vi "FTW-Container-Array-ReplaceSubset.vi"(0 "FTW-Container In":refnum<class "FTW-Container.lvclass">, 7 "Array Elements":refnum<class "FTW-Container.lvclass">[](array[class]), 9 "Index":i32, 11 "error in":errorcluster) -> (4 "FTW-Container Out":refnum<class "FTW-Container.lvclass">, 15 "error out":errorcluster)   [LabVIEW 2015, in "FTW-Container.lvclass"]
uses:
  FTW-Container.lvclass
  FTW-Container.lvclass/FTW-Container.ctl
  <vilib>/Utility/Data Type/NI_Data Type.lvlib
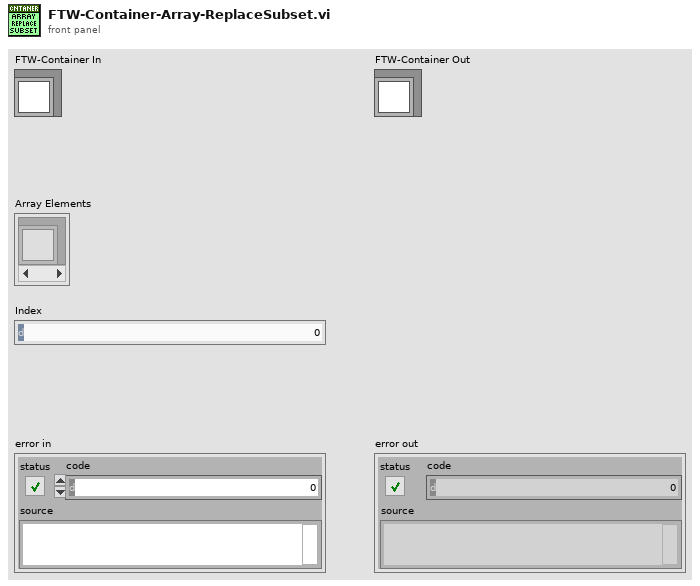
[diagram p1: front panel]
types:
  T1 = typedef "NI_Data Type.lvlib/Data Type.ctl" = enum8{"Invalid Type", "Void", "I8", "I16", "I32", "I64", "U8", "U16", "U32", "U64", "Single Float", "Double Float", "Extended Float", "Single Complex", "Double Complex", "Extended Complex", "Enum U8", "Enum U16", "Enum U32", "Enum U64", "Single Float With Unit", "Double Float With Unit", "Extended Float With Unit", "Single Complex with Unit", "Double Complex with Unit", "Extended Complex with Unit", "Boolean", "String", "Path", "Picture", "Tag", "Array", "Cluster", "Variant", "LV Variant", "Waveform", "Timestamp", "Digital Waveform", "Digital Data", "ExpressData", "Refnum", "External Data", "VI", "Poly VI", "LabVIEW Class Instance", "Fixed Point"}
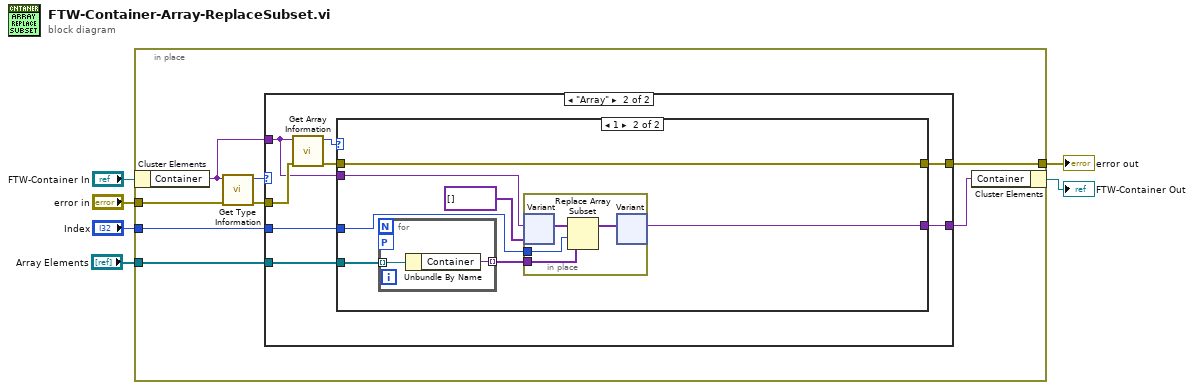
[diagram p0: block diagram]
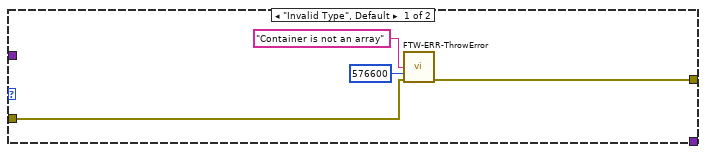
[diagram p2: hidden frame]
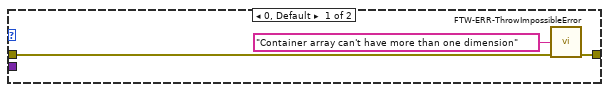
[diagram p3: hidden frame]
diagram:
  n1 = in-place {
    in-place-border: "error in" -> [w14]
    in-place-border: [w12] -> w5
    in-place-border: "Array Elements" -> [w10]
    in-place-border: "Index" -> [w7]
    n2 = in-place-cluster #1("FTW-Container In") -> ("Container"=w9:variant)
    n3 = call <vilib>:"Get Type Information.vi"("error in (no error)"=w14, "Variant"=w9) -> ("error out"=w13:errorcluster, "Type"=w11:T1)  [unwired: 5 in, 3 out]
    n4 = case shown="\"Array\"" w11 {
      tunnel: w13 -> [w18 w24]
      tunnel: [w17 w23] -> w12
      tunnel: w9 -> [_ w22]
      tunnel: w10 -> [_ w21]
      tunnel: [_ w20] -> w8
      tunnel: w7 -> [_ w19]
      frame "Invalid Type", Default {
        n5 = call "FTW-ERR-ThrowError.vi"("Error Message"="Container is not an array", "Error Code"=576600, "error in"=w18) -> ("error out"=w17:errorcluster)  [unwired: 12 in]
      }
      frame "Array" {
        n6 = call <vilib>:"Get Array Information.vi"("error in (no error)"=w24, "Variant"=w22) -> ("error out"=w26:errorcluster, "Number of Dimensions"=w25:i32)  [unwired: 6 in, 2 out]
        n7 = case shown="1" w25 {
          tunnel: w26 -> [w29 w36]
          tunnel: w22 -> [_ w35]
          tunnel: [w28 w36] -> w23
          tunnel: w21 -> [_ w33]
          tunnel: [_ w31] -> w20
          tunnel: w19 -> [_ w30]
          frame 0, Default {
            n8 = call "FTW-ERR-ThrowImpossibleError.vi"("Reason this error should never happen"="Container array can't have more than one dimension", "error in"=w29) -> ("error out"=w28:errorcluster)  [unwired: 13 in]
          }
          frame 1 {
            n9 = for {
              tunnel: w33 -> [w38] mode=indexing
              tunnel: [w37] -> w32 mode=indexing
              workers-P: _ -> [_]
              n10 = Unbundle By Name(w38) -> ("Container"=w37:variant)
            }
            n11 = in-place {
              in-place-border: w32 -> [w40]
              in-place-border: w30 -> [w39]
              n12 = in-place-variant #2(w35, variant[] []) -> (w42:variant[])  [unwired: 1 out]
              n13 = Replace Array Subset(array=w42, new element=w40, index=w39) -> (w41:variant[])
              n14 = in-place-variant #2(w41) -> (w31:variant)  [unwired: 1 out]
            }
          }
        }
      }
    }
    n15 = in-place-cluster #1("Container"=w8) -> (→"FTW-Container Out":refnum<class "FTW-Container.lvclass">)
  }
  "error out" <- w5
